vi "1553B_CMD.vi"(7 "RT地址(默认：10000)":u16=16 format="%.0b", 10 "控制指令子地址(默认：11010":u16=26 format="%.0b", 11 "数据字数组":u16[](array[numeric])) -> (3 "1553B指令":string)   [LabVIEW 2012]
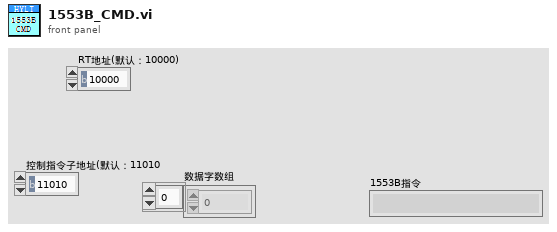
[diagram p1: front panel]
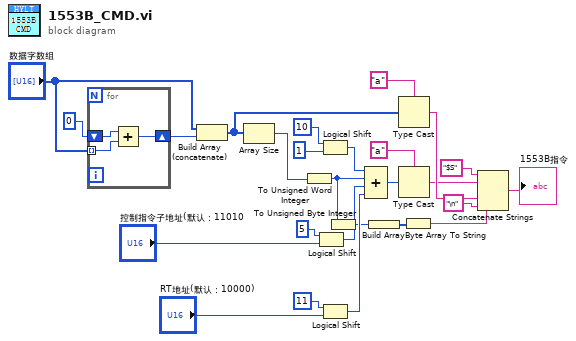
[diagram p0: block diagram]
diagram:
  n1 = for {
    tunnel: "数据字数组" -> [w29] mode=indexing
    shift-right: [w28] -> w6
    shift-left: u16 0 -> [w27]
    n2 = Add(x=w27, y=w29) -> (x+y=w28:u16)
  }
  n3 = Build Array (concatenate)("数据字数组", w6) -> (w5:u16[])
  n4 = Array Size(array=w5) -> (size(s)=w15:i32)
  n5 = To Unsigned Word Integer(number=w15) -> (unsigned 16bit integer=w4:u16)
  n6 = Logical Shift(y=i16 5, x="控制指令子地址(默认：11010") -> (x << y=w21:u16)
  n7 = Logical Shift(y=i16 10, x=u16 1) -> (x << y=w23:u16)
  n8 = Logical Shift(y=i16 11, x="RT地址(默认：10000)") -> (x << y=w17:u16)
  n9 = To Unsigned Byte Integer(number=w4) -> (unsigned 8bit integer=w2:u8)
  n10 = Compound Arithmetic op=ADD(w23, w4, w21, w17) -> (w16:u16)
  n11 = Build Array(w2) -> (w3:u8[])
  n12 = Type Cast(type="a" ("类型"), x=w5) -> (*(type *) &x=w13:string)
  n13 = Type Cast(type="a" ("类型"), x=w16) -> (*(type *) &x=w12:string)
  n14 = Byte Array To String(unsigned byte array=w3) -> (string=w1:string)
  n15 = Concatenate Strings("$S" ("字符串"), w12, w1, w13, "\n" ("字符串")) -> (→"1553B指令":string)
